vi "Select Sheet by Name.vi"(7 "Sheet (Sheet1)":string="Sheet1", 8 "error in (no error)":errorcluster, 11 "Excel Legacy in":refnum<class "Excel Legacy.lvclass">) -> (0 "error out":errorcluster, 3 "Excel Legacy out":refnum<class "Excel Legacy.lvclass">)   [LabVIEW 2013, in "Excel Legacy.lvclass"]
uses:
  Excel Legacy.lvclass
  Spreadsheet.lvclass
  Excel Legacy.lvclass/Excel Legacy.ctl
  C:/PhaeronGit/LVNPOI/Resources/NPOI 2.1.1 dotnet2/NPOI.dll
  Resources/NPOI 2.1.1 dotnet2/NPOI.dll
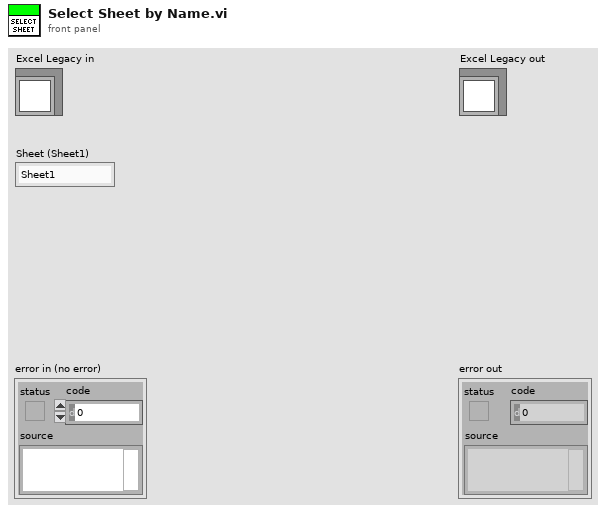
[diagram p1: front panel]
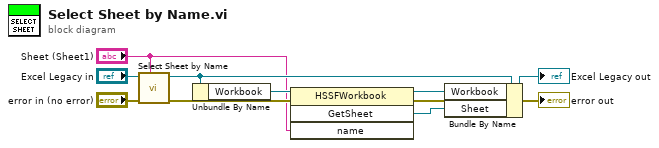
[diagram p0: block diagram]
diagram:
  n1 = call-parent "Select Sheet by Name.vi"("Sheet (Sheet1)"="Sheet (Sheet1)", "error in (no error)"="error in (no error)", "Spreadsheet in"="Excel Legacy in") -> ("error out"=w4:errorcluster, "Spreadsheet out"=w7:refnum<class "Excel Legacy.lvclass">)  [unwired: 7 in]
  n2 = Unbundle By Name(w7) -> ("Workbook"=w6:refnum<k24>)
  n3 = invoke class="HSSFWorkbook" method="GetSheet"(reference=w6, error in=w4, "name"="Sheet (Sheet1)") -> (reference out=w5:refnum<k24>, error out=→"error out":errorcluster, "GetSheet"=w2:refnum<k24>)  [unwired: 1 in, 1 out]
  n4 = Bundle By Name(cluster=w7, "Workbook"=w5, "Sheet"=w2) -> (→"Excel Legacy out":refnum<class "Excel Legacy.lvclass">)
